vi "data analysis.vi"() -> ()   [LabVIEW 2018]
uses:
  <vilib>/ptbypt/NI_PtbyPt.lvlib
  <vilib>/Utility/file.llb/Read Delimited Spreadsheet (string).vi
  <vilib>/Analysis/NI_AALPro.lvlib
  <vilib>/Analysis/2dsp.llb/Real FFT.vi
panel:
  in  "Tab Control":enum32{"Page 1", "Page 2"}(tab)=enum."Page 2"
  in  "file path (dialog if empty)":path
  in  "Enable this function 1":bool
  out "XY Graph":cluster{dbl[], dbl[]}(graph)
  out "Waveform Graph 2":dbl[](graph)
  in  "amplitude":dbl=2.0 format="%0.2f"
  in  "frequency":dbl=20.0 format="%0.2f"
  in  "phase":dbl format="%0.2f"
  in  "time":dbl=0.9999999999999998 format="%0.4f"
  in  "phase 2":dbl format="%0.2f"
  in  "frequency 2":dbl=3.0 format="%0.2f"
  in  "amplitude 2":dbl=1.0 format="%0.2f"
  in  "Counter":i32=3000
  out "FFT(Signal1+2)":cluster{dbl, dbl, dbl[]}(graph)
  out "Signal1&2":cluster{dbl[], dbl[]}[](graph)
  in  "Enable this function 2":bool=TRUE
  out "Signal 1+2":cluster{dbl[], dbl[]}(graph)
  # "Sine"
  # "Cos"
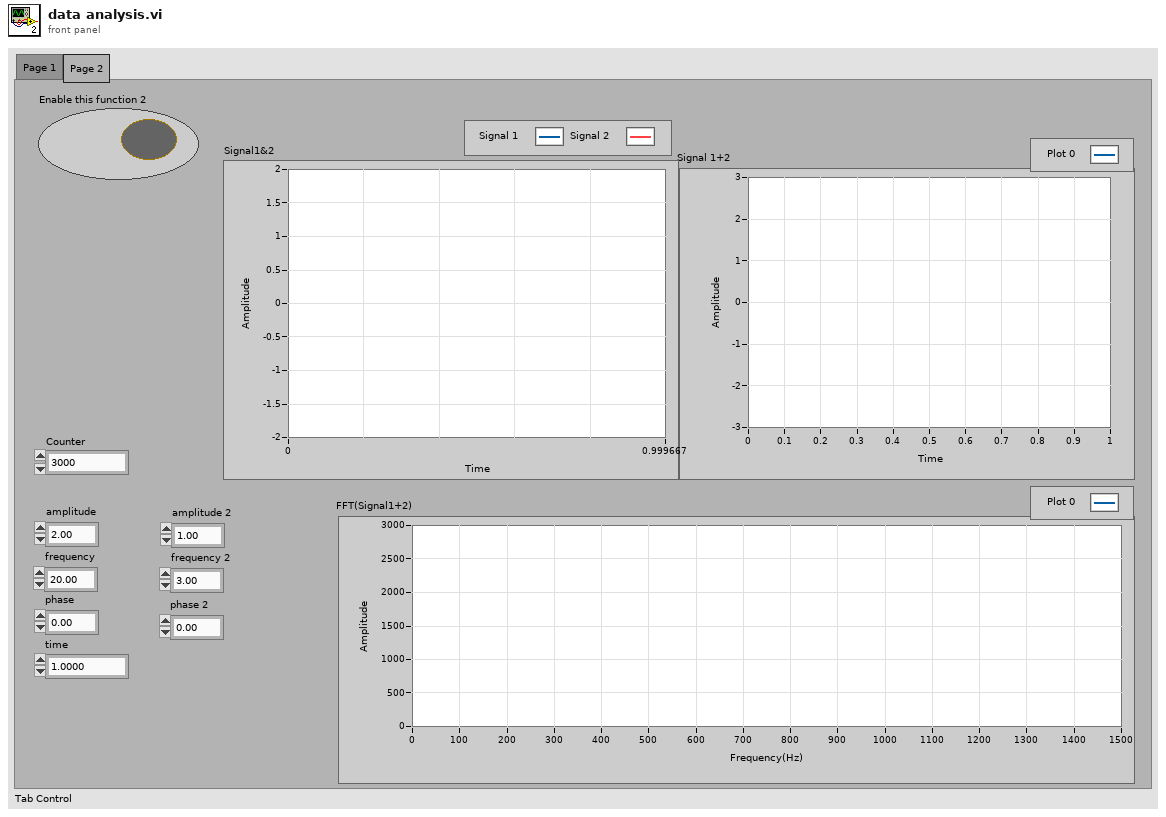
[diagram p1: front panel]
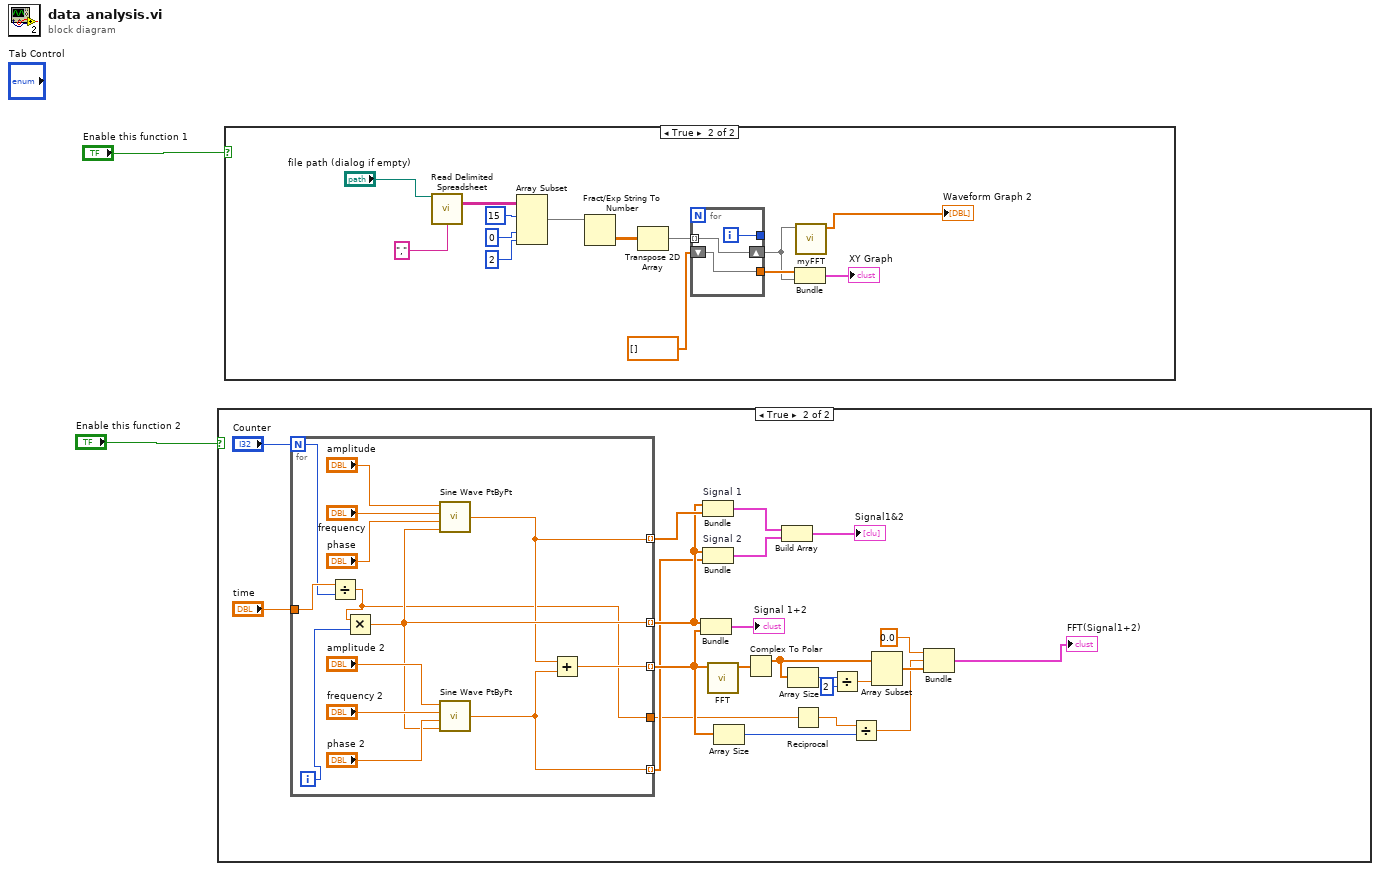
[diagram p0: block diagram]
diagram:
  n1 = case shown="True" "Enable this function 2" {
    frame False {
    }
    frame True {
      n2 = for {
        N: "Counter" -> [w26]
        tunnel: "time" -> [w27]
        tunnel: [w31] -> w16 mode=indexing
        tunnel: [w30] -> w21 mode=indexing
        tunnel: [w29] -> w17 mode=indexing
        tunnel: [w28] -> w15 mode=indexing
        tunnel: [w25] -> w10
        i -> [w32]
        n3 = Divide(x=w27, y=w26) -> (x/y=w25:dbl)
        n4 = Multiply(x=w25, y=w32) -> (x*y=w31:dbl)
        n5 = call <vilib>:"Sine Wave PtByPt.vi"("time"=w31, "phase"="phase", "frequency"="frequency", "amplitude"="amplitude") -> ("sine wave"=w29:dbl)
        n6 = call <vilib>:"Sine Wave PtByPt.vi"("time"=w31, "phase"="phase 2", "frequency"="frequency 2", "amplitude"="amplitude 2") -> ("sine wave"=w28:dbl)
        n7 = Add(x=w29, y=w28) -> (x+y=w30:dbl)
      }
      n8 = Bundle(w16, w21) -> (→"Signal 1+2":cluster{dbl[], dbl[]})  [unwired: 1 in]
      n9 = Bundle "Signal 1"(w16, w17) -> (w14:cluster{dbl[], dbl[]})  [unwired: 1 in]
      n10 = Bundle "Signal 2"(w16, w15) -> (w13:cluster{dbl[], dbl[]})  [unwired: 1 in]
      n11 = call-poly <vilib>:"FFT.vi"("X"=w21) -> ("FFT {X}"=w22:cdb[])  [unwired: 9 in, 1 out]
      n12 = Array Size(array=w21) -> (size(s)=w8:i32)
      n13 = Complex To Polar(r * e^(i*theta)=w22) -> (r=w6:dbl[])  [unwired: 1 out]
      n14 = Build Array(w14, w13) -> (→"Signal1&2":cluster{dbl[], dbl[]}[])
      n15 = Array Size(array=w6) -> (size(s)=w4:i32)
      n16 = Reciprocal(x=w10) -> (1/x=w7:dbl)
      n17 = Divide(x=w4, y=2) -> (x/y=w5:dbl)
      n18 = Divide(x=w7, y=w8) -> (x/y=w9:dbl)
      n19 = Array Subset(array=w6, length=w5) -> (w18:dbl[])  [unwired: 1 in]
      n20 = Bundle(0.0, w9, w18) -> (→"FFT(Signal1+2)":cluster{dbl, dbl, dbl[]})  [unwired: 1 in]
    }
  }
  n21 = case shown="True" "Enable this function 1" {
    frame False {
    }
    frame True {
      n22 = call-poly <vilib>:"Read Delimited Spreadsheet.vi"("file path (dialog if empty)"="file path (dialog if empty)", "delimiter (\\t)"="," ("delimiter (\\t)")) -> ("all rows"=w50:string[][])  [unwired: 8 in, 5 out]
      n23 = Array Subset(array=w50, index (row)=15 ("index"), index (col)=0 ("index"), length (col)=2 ("length")) -> (w46:string[][])  [unwired: 1 in]
      n24 = Fract/Exp String To Number(string=w46) -> (number=w41:dbl[][])  [unwired: 3 in, 1 out]
      n25 = Transpose 2D Array(2D array=w41) -> (transposed array=w42:dbl[][])
      n26 = for {
        tunnel: w42 -> [w54] mode=indexing
        shift-right: [w54] -> w40
        shift-left: dbl[] [] -> [w55]
        tunnel: [w55] -> w45
        tunnel: [w53] -> _
        i -> [w53]
      }
      n27 = Bundle(w45, w40) -> (→"XY Graph":cluster{dbl[], dbl[]})  [unwired: 1 in]
      n28 = call "myFFT.vi"("Array in"=w40) -> ("FFT {X}"=→"Waveform Graph 2":cdb[])  [unwired: 9 in, 1 out]
    }
  }
